vi "Agilent SNA Set Averaging Factor.vi"(6 "Channel":i8=1 min=1 max=99 step=1, 7 "Agilent SNA":T1, 8 "error in (no error)":errorcluster, 10 "Averaging Factor":i32, 11 "VISA Resource Names":T2) -> (0 "error out":errorcluster, 3 "dup VISA Resource Names":T2)   [LabVIEW 2011]
doc: "This vi sets the power range. Only works on the HP 8753D."
uses:
  TypeDefs/Agilent SNA VISA.ctl
  TypeDefs/Agilent SNA Instrument Info.ctl
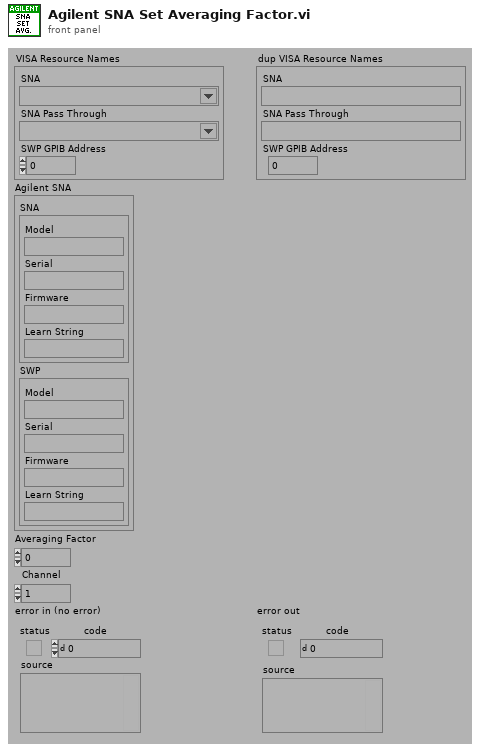
[diagram p1: front panel]
types:
  T1 = typedef "Agilent SNA Instrument Info.ctl" = cluster{"SNA":cluster{"Model":string, "Serial":string, "Firmware":string, "Learn String":string}, "SWP":cluster{"Model":string, "Serial":string, "Firmware":string, "Learn String":string}}
  T2 = typedef "Agilent SNA VISA.ctl" = cluster{"SNA":refnum<visa-resource-name>, "SNA Pass Through":refnum<visa-resource-name>, "SWP GPIB Address":i32}
  T3 = typedef "Agilent SNA Model.ctl" = enum16{"Not Supported", "8757X"}
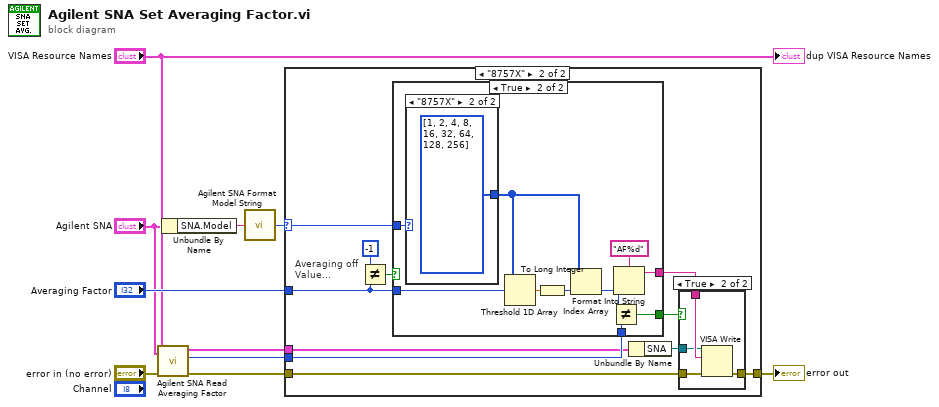
[diagram p0: block diagram]
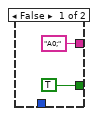
[diagram p3: hidden frame]
diagram:
  n1 = call "Agilent SNA Read Averaging Factor.vi"("Agilent SNA"="Agilent SNA", "error in (no error)"="error in (no error)", "VISA Resource Names"="VISA Resource Names") -> ("error out"=w8:errorcluster, "Averaging Factor"=w7:i32, "dup VISA Resource Names"=w2:T2)  [unwired: 1 in, 5 out]
  n2 = Unbundle By Name("Agilent SNA") -> ("SNA.Model"=w4:string)
  n3 = call "Agilent SNA Format Model String.vi"("Model String"=w4) -> ("Model"=w5:T3)
  n4 = case shown="\"8757X\"" w5 {
    selector: w5 -> [_ w18]
    tunnel: [w11 w22] -> w10
    tunnel: w8 -> [w11 w21]
    tunnel: w2 -> [_ w16]
    tunnel: w7 -> [_ w20]
    tunnel: "Averaging Factor" -> [_ w13]
    frame "Not Supported" {
    }
    frame "8757X" {
      # "Averaging off \nValue..."
      n5 = Not Equal?(x=-1 ("y"), y=w13) -> (x != y?=w14:bool)
      n6 = case shown="True" w14 {
        tunnel: w20 -> [_ w34]
        tunnel: [TRUE w33] -> w19
        tunnel: w18 -> [_ w32]
        tunnel: ["A0;" w30] -> w17
        tunnel: w13 -> [_ w26]
        frame False {
        }
        frame True {
          n7 = case shown="\"8757X\"" w32 {
            tunnel: [_ i32[] [1, 2, 4, 8, 16, 32, 64, 128, 256]] -> w27
            frame "Not Supported" {
            }
            frame "8757X" {
            }
          }
          n8 = Threshold 1D Array(2:w26, 3:w27) -> (0:w28:dbl)  [unwired: 1 out]
          n9 = To Long Integer(number=w28) -> (32bit integer=w29:i32)
          n10 = Index Array(array=w27, index=w29) -> (element=w25:i32)
          n11 = Not Equal?(x=w25, y=w34) -> (x != y?=w33:bool)
          n12 = Format Into String(format string="AF%d", w25) -> (resulting string=w30:string)  [unwired: 2 in, 1 out]
        }
      }
      n13 = Unbundle By Name(w16) -> ("SNA"=w15:refnum<visa-resource-name>)
      n14 = case shown="True" w19 {
        tunnel: [w36 w40] -> w22
        tunnel: w17 -> [_ w39]
        tunnel: w21 -> [w36 w37]
        tunnel: w15 -> [_ w38]
        frame False {
        }
        frame True {
          n15 = VISA Write(VISA resource name=w38, write buffer=w39, error in (no error)=w37) -> (error out=w40:errorcluster)  [unwired: 2 out]
        }
      }
    }
  }
  "error out" <- w10
  "dup VISA Resource Names" <- "VISA Resource Names"
